vi "Joystick_Globals.vi"() -> ()   [LabVIEW 2019]
panel:
  in  "Copilot_Joystick":string="Copilot_Joystick"
  in  "Pilot_Joystick":string="Pilot_Joystick"
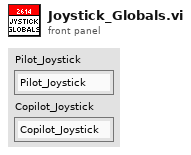
[diagram p1: front panel]
diagram:
